vi "Follow Polynomial (aka the DREAM).vi"() -> ()   [LabVIEW 2015]
uses:
  <vilib>/Rock Robotics/WPI/CAN/TalonSRX/WPI_CANTalonSRX_APIControlMode.ctl
  <vilib>/addons/control/pid/NI_PID_pid.lvlib
  <vilib>/addons/control/pid/pid.llb/PID (DBL).vi
  Polynomial First Derivitive.vi
  <vilib>/Rock Robotics/WPI/CAN/Jaguar/SubVIs/WPI_CANJaguar_ControlMode.ctl
  <vilib>/Rock Robotics/SystemInterfaces/DIO/FPGA_DIOPWMChannel.ctl
  <vilib>/Rock Robotics/WPI/PWM/WPI_PWMDeadband.ctl
  <vilib>/Rock Robotics/WPI/MotorControl/WPI_MotorControlType.ctl
  <vilib>/Rock Robotics/WPI/MotorControl/WPI_MotorControlDeviceRef.ctl
panel:
  in  "Right bound":dbl
  in  "Ticks Per Foot":dbl
  in  "Current Mode":dbl
  in  "Motor Refs":T1[](array[typedef])
  in  "PID Distance gains":T8={"proportional gain (Kc)"=1.0, "integral time (Ti, min)"=0.01, "derivative time (Td, min)"=0.0} {"derivative time (Td, min)" format="%.3f"; "integral time (Ti, min)" format="%.3f"; "proportional gain (Kc)" format="%.3f"}
  in  "Angle Tolerance":dbl=2.0
  in  "Max Turn Speed":dbl
  in  "Polynomial":dbl[](array[numeric])
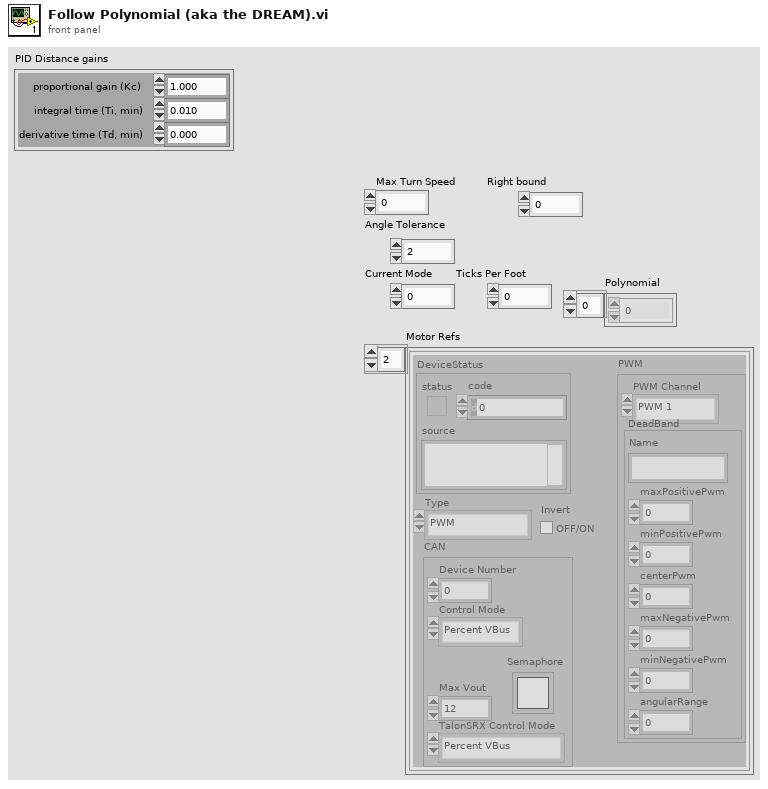
[diagram p1: front panel]
types:
  T1 = typedef "WPI_MotorControlDeviceRef.ctl" = cluster{"DeviceStatus":errorcluster, "Type":T2, "PWM":cluster{"PWM Channel":T3, "DeadBand":T4}, "CAN":cluster{"Device Number":u8, "Control Mode":T5, "Semaphore":T6, "Max Vout":dbl, "TalonSRX Control Mode":T7}, "Invert":bool}
  T2 = typedef "WPI_MotorControlType.ctl" = enum16{"PWM", "CAN", "CANTalonSRX"}
  T3 = typedef "FPGA_DIOPWMChannel.ctl" = enum8{"PWM 0", "PWM 1", "PWM 2", "PWM 3", "PWM 4", "PWM 5", "PWM 6", "PWM 7", "PWM 8", "PWM 9", "PWM MXP 0", "PWM MXP 1", "PWM MXP 2", "PWM MXP 3", "PWM MXP 4", "PWM MXP 5", "PWM MXP 6", "PWM MXP 7", "PWM MXP 8", "PWM MXP 9", "Invalid"}
  T4 = typedef "WPI_PWMDeadband.ctl" = cluster{"Name":string, "maxPositivePwm":i32, "minPositivePwm":i32, "centerPwm":i32, "maxNegativePwm":i32, "minNegativePwm":i32, "angularRange":u16}
  T5 = typedef "WPI_CANJaguar_ControlMode.ctl" = enum8{"Percent VBus", "Current", "Speed", "Position", "Voltage"}
  T6 = typedef "Semaphore RefNum" = refnum<k1>
  T7 = typedef "WPI_CANTalonSRX_APIControlMode.ctl" = enum8{"Percent VBus", "Speed", "Position", "Slave", "Unchanged / Invalid", "Voltage Compensation", "Current", "Motion Profile"}
  T8 = cluster{"proportional gain (Kc)":dbl, "integral time (Ti, min)":dbl, "derivative time (Td, min)":dbl}
  T9 = typedef "WPI_CANTalonSRX_GlobalStatus.ctl" = cluster{"Applied Throttle":dbl, "Module Enabled":bool, "CAN Error":errorcluster, "Closed Loop Error":dbl, "Forward Limit Switch Closed":bool, "Reverse Limit Switch Closed":bool, "Sensor Position":dbl, "Sensor Velocity":dbl, "Current":dbl, "Sticky Fault - Over Temp":bool, "Sticky Fault - Under Voltage":bool, "Sticky Fault - Forward Limit":bool, "Sticky Fault - Reverse Limit":bool, "Sticky Fault - Forward Soft Limit":bool, "Sticky Fault - Reverse Soft Limit":bool, "Brake is Enabled":bool, "Encoder Position":dbl, "Encoder Velocity":dbl, "Encoder Index Count":dbl, "Encoder A Pin State":bool, "Encoder B Pin State":bool, "Encoder Index Pin State":bool, "Analog In":dbl, "Analog In Velocity":dbl, "Temperature (C)":dbl, "Battery Voltage":dbl, "Control 5 Is Supported":bool, "Current Profile Slot Select":dbl, "Pos Div 8":bool, "Vel Div 4":bool, "Pulse Width Position":i32, "Pulse Width Velocity":i32, "Pulse Width Rise To Rise (us)":i32, "Pulse Width Rise To Fall (us)":i32, "Mot Prof Active Is Under Run":bool, "Mot Prof Active Has Under Run":bool, "Mot Prof Active Is Last":bool, "Mot Prof Active Velocity Only":bool, "Mot Prof Active Is Valid":bool, "Mot Prof Buffer Is Full":bool, "Mot Prof Active Profile Slot Select":i32, "Mot Prof NextID":i32, "Mot Prof Count":i32, "Mot Prof Active Velocity":dbl, "Mot Prof Active Position":dbl, "Mot Prof Output Enable":i32}
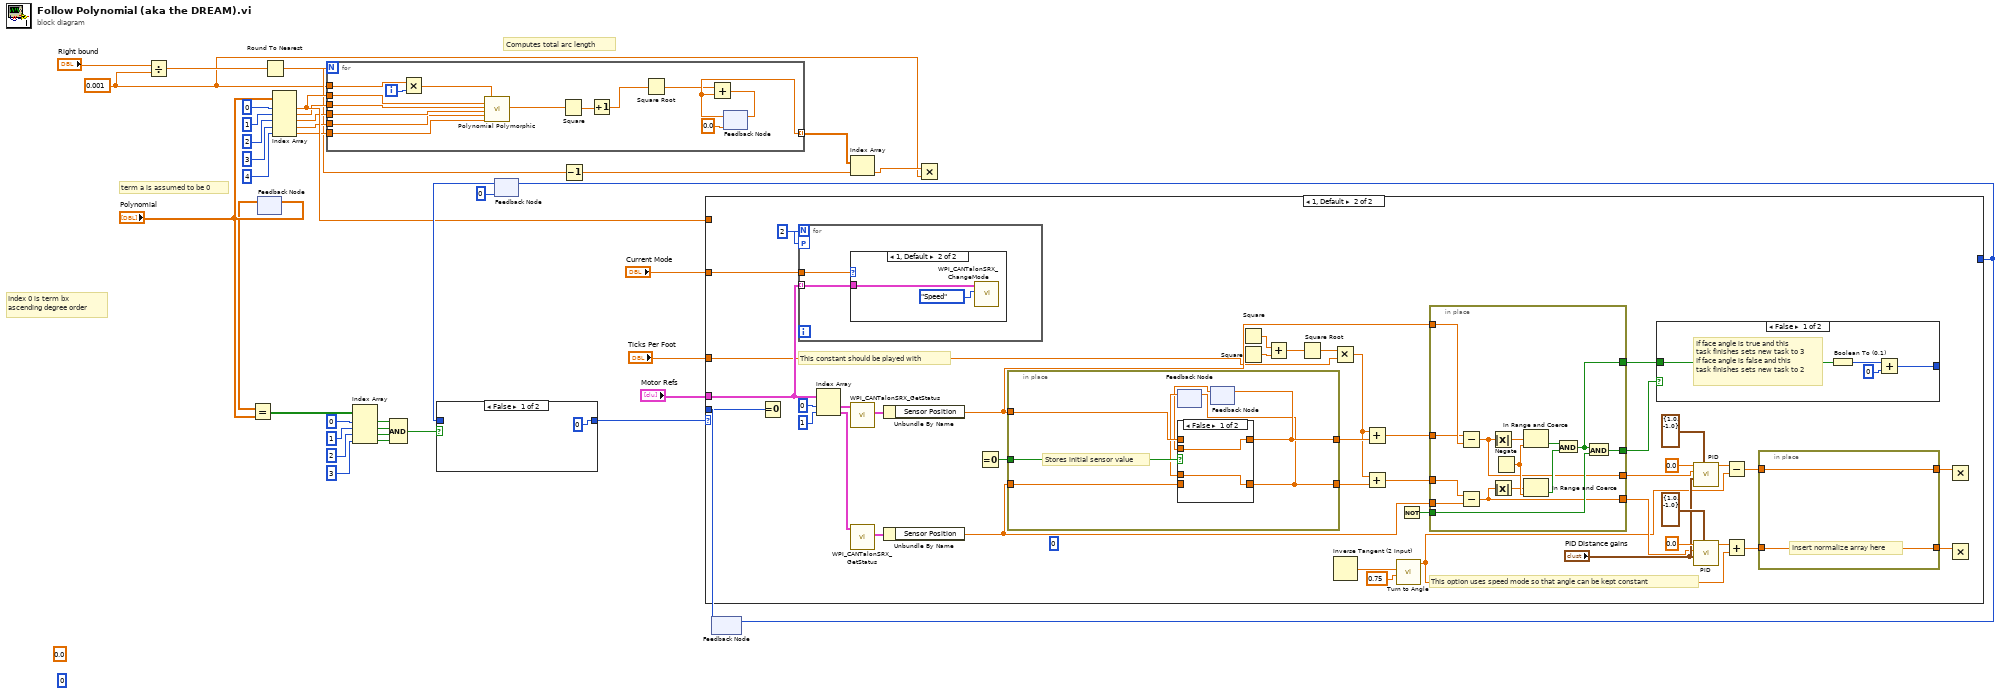
[diagram p0: block diagram]
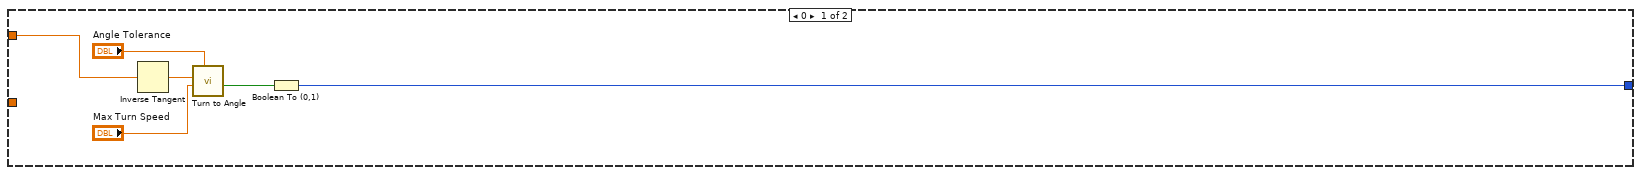
[diagram p3: hidden frame]
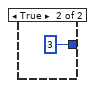
[diagram p4: hidden frame]
diagram:
  w1 = 0.001
  (unwired) 0.0 ("a")
  (unwired) 0 ("index")
  # "Computes total arc length"
  # "term a is assumed to be 0"
  # "Index 0 is term bx \nascending degree order"
  n1 = Divide(x="Right bound", y=w1) -> (x/y=w12:dbl)
  n2 = feedback-in #1("Polynomial") -> ()
  n3 = feedback #1() -> (w32:dbl[])  [unwired: 1 in]
  n4 = Equal?(x=w32, y="Polynomial") -> (x = y?=w28:bool[])
  n5 = Round To Nearest(number=w12) -> (nearest integer value=w4:dbl)
  n6 = Index Array(array="Polynomial", index #1=0 ("index"), index #2=1 ("index"), index #3=2 ("index"), index #4=3 ("index"), index #5=4) -> (element #1=w11:dbl, element #2=w10:dbl, element #3=w9:dbl, element #4=w7:dbl, element #5=w6:dbl)
  n7 = for {
    N: w4 -> [_]
    tunnel: w11 -> [w52]
    tunnel: w10 -> [w51]
    tunnel: w9 -> [w50]
    tunnel: w7 -> [w49]
    tunnel: w6 -> [w48]
    tunnel: w1 -> [w46]
    tunnel: [w42] -> w5 mode=indexing
    i -> [w47]
    n8 = Multiply(x=w46, y=w47) -> (x*y=w45:dbl)
    n9 = call-poly "Polynomial Polymorphic.vi"("BX"=w52, "CX^2"=w51, "DX^3"=w50, "EX^4"=w49, "FX^5"=w48, "X"=w45) -> ("Y"=w41:dbl)  [unwired: 13 in]
    n10 = Square(x=w41) -> (x^2=w40:dbl)
    n11 = Increment(x=w40) -> (x+1=w39:dbl)
    n12 = Square Root(x=w39) -> (sqrt(x)=w38:dbl)
    n13 = feedback #2(0.0) -> (w42:dbl)
    n14 = Add(x=w38, y=w42) -> (x+y=w44:dbl)
    n15 = feedback-in #2(w44) -> ()
  }
  n16 = Index Array(array=w28, index #1=0 ("index"), index #2=1 ("index"), index #3=2 ("index"), index #4=3 ("index")) -> (element #1=w27:bool, element #2=w26:bool, element #3=w25:bool, element #4=w24:bool)
  n17 = Compound Arithmetic op=AND(w27, w26, w25, w24) -> (w23:bool)
  n18 = feedback #3(0) -> (w20:i32)
  n19 = case shown="False" w23 {
    tunnel: [0 w54] -> w21
    tunnel: w20 -> [_ w54]
    frame False {
    }
    frame True {
    }
  }
  n20 = Decrement(x=w4) -> (x-1=w3:dbl)
  n21 = feedback #4() -> (w18:i16)  [unwired: 1 in]
  n22 = case shown="1, Default" w21 {
    tunnel: w11 -> [w60 _]
    tunnel: [w55 _] -> w19
    tunnel: w18 -> [_ w102]
    tunnel: "Motor Refs" -> [_ w63]
    tunnel: "Current Mode" -> [_ w62]
    tunnel: "Ticks Per Foot" -> [_ w61]
    frame 0 {
      n23 = Inverse Tangent(1:w60) -> (0:w59:dbl)
      n24 = call "Turn to Angle.vi"("Angle Tolerance"="Angle Tolerance", "Rotation Multiplier"="Max Turn Speed", "Target angle"=w59) -> ("Finished?"=w56:bool)  [unwired: 4 in, 1 out]
      n25 = Boolean To (0,1)(Boolean=w56) -> (0, 1=w55:i16)
    }
    frame 1, Default {
      w97 = 2
      (unwired) 0
      # "This constant should be played with"
      # "This option uses speed mode so that angle can be kept constant"
      n26 = Equal To 0?(x=w102) -> ()  [unwired: 1 out]
      n27 = for {
        N: w97 -> [_]
        tunnel: w63 -> [w136] mode=indexing
        tunnel: w62 -> [w135]
        workers-P: w97 -> [_]
        n28 = case shown="1, Default" w135 {
          tunnel: w136 -> [_ w138]
          frame 0 {
          }
          frame 1, Default {
            n29 = call <vilib>:"WPI_CANTalonSRX_ChangeMode.vi"("Control Mode"=WPI_CANTalonSRX_APIControlMode."Speed", "CAN Talon SRX Ref"=w138) -> ()  [unwired: 8 in, 2 out]
          }
        }
      }
      n30 = Index Array(array=w63, index #1=0 ("index"), index #2=1 ("index")) -> (element #1=w92:T1, element #2=w90:T1)
      n31 = call <vilib>:"WPI_CANTalonSRX_GetStatus.vi"("CAN Talon SRX Ref"=w92) -> ("Talon SRX Status"=w91:T9)  [unwired: 8 in, 2 out]
      n32 = call <vilib>:"WPI_CANTalonSRX_GetStatus.vi"("CAN Talon SRX Ref"=w90) -> ("Talon SRX Status"=w89:T9)  [unwired: 8 in, 2 out]
      n33 = Unbundle By Name(w91) -> ("Sensor Position"=w78:dbl)
      n34 = Unbundle By Name(w89) -> ("Sensor Position"=w85:dbl)
      n35 = Equal To 0?() -> (x = 0?=w95:bool)  [unwired: 1 in]
      n36 = in-place {
        in-place-border: w95 -> [w130]
        in-place-border: w78 -> [w129]
        in-place-border: w85 -> [w128]
        in-place-border: [w127] -> w88
        in-place-border: [w124] -> w86
        # "Stores initial sensor value"
        n37 = feedback #5() -> (w126:dbl)  [unwired: 1 in]
        n38 = feedback #6() -> (w125:dbl)  [unwired: 1 in]
        n39 = case shown="False" w130 {
          tunnel: [w132 w134] -> w127
          tunnel: w129 -> [_ w134]
          tunnel: w125 -> [w132 _]
          tunnel: [w131 w133] -> w124
          tunnel: w128 -> [_ w133]
          tunnel: w126 -> [w131 _]
          frame False {
          }
          frame True {
          }
        }
        n40 = feedback-in #5(w124) -> ()
        n41 = feedback-in #6(w127) -> ()
      }
      n42 = Square() -> (x^2=w100:dbl)  [unwired: 1 in]
      n43 = Square() -> (x^2=w101:dbl)  [unwired: 1 in]
      n44 = Add(x=w100, y=w101) -> (x+y=w99:dbl)
      n45 = Square Root(x=w99) -> (sqrt(x)=w98:dbl)
      n46 = Multiply(x=w98, y=w61) -> (x*y=w87:dbl)
      n47 = Inverse Tangent (2 Input)() -> (0:w72:dbl)  [unwired: 2 in]
      n48 = Add(x=w87, y=w88) -> (x+y=w79:dbl)
      n49 = Add(x=w87, y=w86) -> (x+y=w82:dbl)
      n50 = call "Turn to Angle.vi"("Rotation Multiplier"=0.75, "Target angle"=w72) -> ("Turn Set Point"=w71:dbl)  [unwired: 5 in, 1 out]
      n51 = Not() -> (.not. x?=w96:bool)  [unwired: 1 in]
      n52 = in-place {
        in-place-border: w96 -> [w118]
        in-place-border: w85 -> [w108]
        in-place-border: w82 -> [w107]
        in-place-border: w78 -> [w106]
        in-place-border: w79 -> [w105]
        in-place-border: [w112] -> w83
        in-place-border: [w111] -> w84
        in-place-border: [w110] -> w77
        in-place-border: [w109] -> w73
        n53 = Subtract(x=w105, y=w106) -> (x-y=w110:dbl)
        n54 = Subtract(x=w107, y=w108) -> (x-y=w109:dbl)
        n55 = Absolute Value(x=w110) -> (abs(x)=w116:dbl)
        n56 = Absolute Value(x=w109) -> (abs(x)=w115:dbl)
        n57 = Negate() -> (-x=w117:dbl)  [unwired: 1 in]
        n58 = In Range and Coerce(x=w116, lower limit=w117) -> (In Range?=w114:bool)  [unwired: 1 in, 1 out]
        n59 = In Range and Coerce(x=w115, lower limit=w117) -> (In Range?=w113:bool)  [unwired: 1 in, 1 out]
        n60 = And(x=w114, y=w113) -> (x .and. y?=w111:bool)
        n61 = And(x=w111, y=w118) -> (x .and. y?=w112:bool)
      }
      n62 = case shown="False" w83 {
        tunnel: [w119 3] -> _
        tunnel: w84 -> [w122 _]
        frame False {
          # "If face angle is true and this \ntask finishes sets new task to 3\nIf face angle is false and this \ntask finishes sets new task to 2"
          n63 = Boolean To (0,1)(Boolean=w122) -> (0, 1=w121:i16)
          n64 = Add(x=w121, y=0) -> (x+y=w119:i32)
        }
        frame True {
        }
      }
      n65 = call-poly <vilib>:"PID.vi"("output range"=cluster{"output high":dbl, "output low":dbl} {"output high"=1.0, "output low"=-1.0}, "PID gains"="PID Distance gains", "process variable"=w77, "setpoint"=0.0) -> ("output"=w69:dbl)  [unwired: 6 in, 1 out]
      n66 = call-poly <vilib>:"PID.vi"("output range"=cluster{"output high":dbl, "output low":dbl} {"output high"=1.0, "output low"=-1.0}, "PID gains"="PID Distance gains", "process variable"=w73, "setpoint"=0.0) -> ("output"=w68:dbl)  [unwired: 6 in, 1 out]
      n67 = Subtract(x=w69, y=w71) -> (x-y=w67:dbl)
      n68 = Add(x=w68, y=w71) -> (x+y=w64:dbl)
      n69 = in-place {
        in-place-border: w67 -> [w104]
        in-place-border: [w104] -> w66
        in-place-border: [w103] -> w65
        in-place-border: w64 -> [w103]
        # "Insert normalize array here"
      }
      n70 = Multiply(x=w66) -> ()  [unwired: 1 in, 1 out]
      n71 = Multiply(x=w65) -> ()  [unwired: 1 in, 1 out]
    }
  }
  n72 = feedback-in #3(w19) -> ()
  n73 = feedback-in #4(w19) -> ()
  n74 = Index Array(array=w5, index=w3) -> (element=w2:dbl)
  n75 = Multiply(x=w2, y=w1) -> ()  [unwired: 1 out]
